vi "test Verify g-cli.vi"(8 "error in":errorcluster, 11 "Test Case In":refnum<class "LUnit Extensions Tests.lvclass">) -> (0 "error out":errorcluster, 3 "Test Case Out":refnum<class "LUnit Extensions Tests.lvclass">)   [LabVIEW 2025, in "LUnit Extensions Tests.lvclass"]
uses:
  LUnit Extensions Tests.lvclass
  C:/Program Files/National Instruments/LabVIEW 2026/vi.lib/Astemes/LUnit/Test Case.lvclass
  Source/Extensions/LUnit.Extension/LUnit.Extension.lvlib
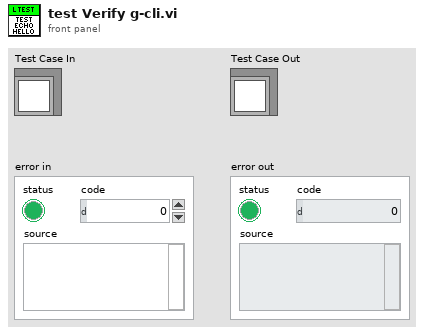
[diagram p1: front panel]
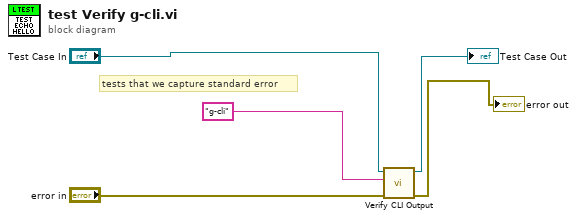
[diagram p0: block diagram]
diagram:
  # "tests that we capture standard error"
  n1 = call "Verify CLI Output.vi"("error in"="error in", "command line"="g-cli", "LUnit Test Case In"="Test Case In") -> ("error out"=→"error out":errorcluster, "LUnit Test Case Out"=→"Test Case Out":refnum<class "LUnit Extensions Tests.lvclass">)  [unwired: 7 in]
